vi "Write.vi"(10 "Double":dbl, 11 "Double in":refnum<class "Double.lvclass">) -> (3 "Double out":refnum<class "Double.lvclass">)   [LabVIEW 2020, in "Data.lvlib" / "Double.lvclass"]
doc: "Write Double."
uses:
  Double.lvclass
  Double.lvclass/Double.ctl
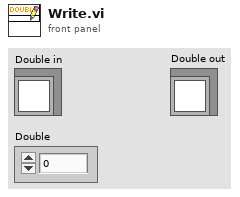
[diagram p1: front panel]
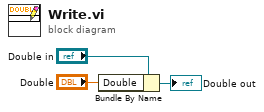
[diagram p0: block diagram]
diagram:
  n1 = Bundle By Name(cluster="Double in", "Double"="Double") -> (→"Double out":refnum<class "Double.lvclass">)
